vi "Local Configuration.INTCSR.Local Interrupt Input Enable.Set.vi"(8 "error in (no error)":errorcluster, 10 "Enable Local Interrupt Input?":bool, 11 "GE 5565PIORC":refnum<class "GE 5565PIORC Old.lvclass">) -> (0 "error out":errorcluster, 3 "GE 5565PIORC out":refnum<class "GE 5565PIORC Old.lvclass">)   [LabVIEW 2016, in "GE 5565PIORC Old.lvclass"]
uses:
  GE 5565PIORC Old.lvclass
  Controls/Registers.Local Configuration.ctl
  GE 5565PIORC Old.lvclass/GE 5565PIORC Old.ctl
  <vilib>/Instr/_visa.llb/VISA Register Access Address Space.ctl
  Binary Operations/Set Bits U32.vi
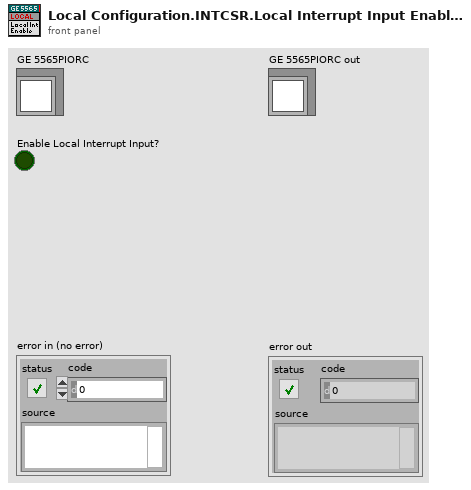
[diagram p1: front panel]
types:
  T1 = typedef "GE 5565PIORC Old.lvclass/Registers.Local Configuration.ctl" = enum16{"DMA Arbitration", "Interrupt Control and Status", "DMA Mode", "DMA PCI Address", "DMA Local Address", "DMA Transfer Size", "DMA Descriptor Pointer", "DMA Command/Status", "DMA PCI DAC Upper Address", "PCI PIO Address Range", "PCI PIO Base Address (Remap)"}
  T2 = typedef "VISA Register Access Address Space.ctl" = u16
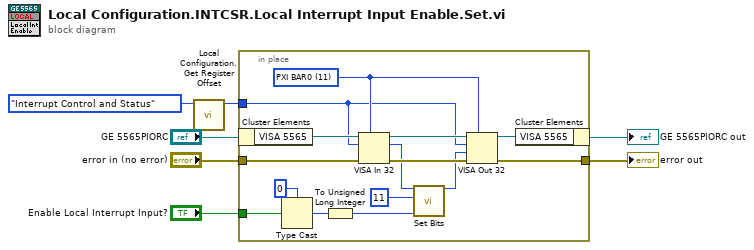
[diagram p0: block diagram]
diagram:
  n1 = call "Local Configuration.Get Register Offset.vi"("Local Configuration Register"=Registers.Local_Configuration."Interrupt Control and Status" ("Local Configration Register Offset")) -> ("Offset"=w1:u32)  [unwired: 10 in]
  n2 = in-place {
    in-place-border: "error in (no error)" -> [w21]
    in-place-border: [w17] -> w5
    in-place-border: "Enable Local Interrupt Input?" -> [w10]
    in-place-border: w1 -> [w8]
    w14 = T2 11 items=["VXI/VME A16"=1, "VXI/VME A24"=2, "VXI/VME A32"=3, "VXI/VME A64"=4, "PXI Memory Allocations"=9, "PXI Configuration"=10, "PXI BAR0"=11, "PXI BAR1"=12, "PXI BAR2"=13, "PXI BAR3"=14, "PXI BAR4"=15, "PXI BAR5"=16] ("Address Space")
    n3 = in-place-cluster #1("GE 5565PIORC") -> ("VISA 5565"=w22:refnum<visa-resource-name>)
    n4 = Type Cast(type=u8 0 ("Start Index (0)"), x=w10) -> (*(type *) &x=w11:u8)
    n5 = To Unsigned Long Integer(number=w11) -> (unsigned 32bit integer=w9:u32)
    n6 = VISA In 32(7:w14, 8:w21, 10:w8, 11:w22) -> (0:w19:errorcluster, 2:w15:u32, 3:w20:refnum<visa-resource-name>)
    n7 = call-poly "Set Bits.vi"("Value (0)"=w9, "Start Index (0)"=u8 11, "Register in"=w15) -> ("Register out"=w16:u32)  [unwired: 6 in, 2 out]
    n8 = VISA Out 32(7:w14, 8:w19, 9:w16, 10:w8, 11:w20) -> (0:w17:errorcluster, 3:w18:refnum<visa-resource-name>)
    n9 = in-place-cluster #1("VISA 5565"=w18) -> (→"GE 5565PIORC out":refnum<class "GE 5565PIORC Old.lvclass">)
  }
  "error out" <- w5
